vi "Update-status-leds.vi"(8 "error in (no error)":errorcluster, 11 "Module status in":T1) -> (0 "error out":errorcluster, 3 "Module status":T1)   [LabVIEW 2013, in "CameraVision.lvlib" / "CV-UI.lvclass"]
uses:
  CV-UI.lvclass
  Status-overview.ctl
  Module-states.ctl
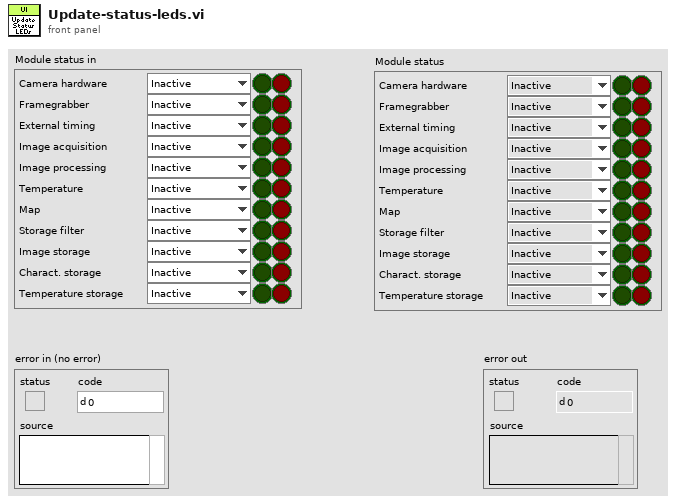
[diagram p1: front panel]
types:
  T1 = typedef "CameraVision.lvlib/CV-UI.lvclass/Status-overview.ctl" = cluster{"Camera hardware":T2, "Framegrabber":T2, "External timing":T2, "Image acquisition":T2, "Image processing ":T2, "Temperature":T2, "Map":T2, "Storage filter":T2, "Image storage":T2, "Charact. storage":T2, "Temperature storage":T2, "Camera hardware G":bool, "Camera hardware R":bool, "Framegrabber G":bool, "Framegrabber R":bool, "External timing G":bool, "External timing R":bool, "Image acquisition G":bool, "Image acquisition R":bool, "Image processing G":bool, "Image processing R":bool, "Temperature G":bool, "Temperature R":bool, "Map G":bool, "Map R":bool, "Storage filter G":bool, "Storage filter R":bool, "Image storage G":bool, "Image storage R":bool, "Charact storage G":bool, "Charact storage R":bool, "Temperature storage G":bool, "Temperature storage R":bool}
  T2 = typedef "CameraVision.lvlib/CV-UI.lvclass/Module-states.ctl" = enum16{"Inactive", "Active", "Data-loss", "Error", "Simulation", "Synchronizing", "Initialized", "Released"}
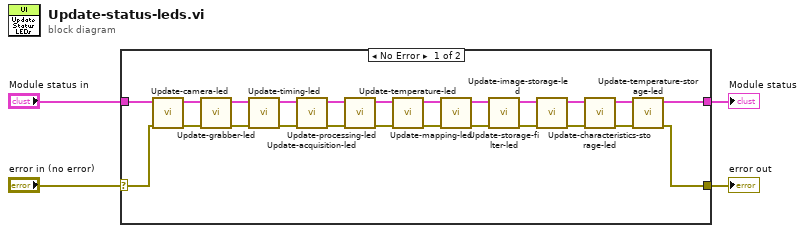
[diagram p0: block diagram]
diagram:
  n1 = case shown="No Error" "error in (no error)" {
    selector: "error in (no error)" -> [w16 w30]
    tunnel: [w15 w30] -> w3
    tunnel: "Module status in" -> [w28 w29]
    tunnel: [w17 w29] -> w1
    frame No Error {
      n2 = call "Update-camera-led.vi"("error in (no error)"=w16, "Module status in"=w28) -> ("error out"=w14:errorcluster, "Module status"=w27:T1)  [unwired: 8 in]
      n3 = call "Update-grabber-led.vi"("error in (no error)"=w14, "Module status in"=w27) -> ("error out"=w13:errorcluster, "Module status"=w26:T1)  [unwired: 8 in]
      n4 = call "Update-timing-led.vi"("error in (no error)"=w13, "Module status in"=w26) -> ("error out"=w12:errorcluster, "Module status"=w25:T1)  [unwired: 8 in]
      n5 = call "Update-acquisition-led.vi"("error in (no error)"=w12, "Module status in"=w25) -> ("error out"=w11:errorcluster, "Module status"=w24:T1)  [unwired: 8 in]
      n6 = call "Update-processing-led.vi"("error in (no error)"=w11, "Module status in"=w24) -> ("error out"=w10:errorcluster, "Module status"=w23:T1)  [unwired: 8 in]
      n7 = call "Update-temperature-led.vi"("error in (no error)"=w10, "Module status in"=w23) -> ("error out"=w9:errorcluster, "Module status"=w22:T1)  [unwired: 8 in]
      n8 = call "Update-mapping-led.vi"("error in (no error)"=w9, "Module status in"=w22) -> ("error out"=w8:errorcluster, "Module status"=w21:T1)  [unwired: 8 in]
      n9 = call "Update-storage-filter-led.vi"("error in (no error)"=w8, "Module status in"=w21) -> ("error out"=w7:errorcluster, "Module status"=w20:T1)  [unwired: 8 in]
      n10 = call "Update-image-storage-led.vi"("error in (no error)"=w7, "Module status in"=w20) -> ("error out"=w6:errorcluster, "Module status"=w19:T1)  [unwired: 8 in]
      n11 = call "Update-characteristics-storage-led.vi"("error in (no error)"=w6, "Module status in"=w19) -> ("error out"=w5:errorcluster, "Module status"=w18:T1)  [unwired: 8 in]
      n12 = call "Update-temperature-storage-led.vi"("error in (no error)"=w5, "Module status in"=w18) -> ("error out"=w15:errorcluster, "Module status"=w17:T1)  [unwired: 8 in]
    }
    frame Error {
    }
  }
  "Module status" <- w1
  "error out" <- w3
